vi "Target Get Gaussian Torque Setpoint.vi"(11 "Phase":dbl) -> (3 "Setpoint":dbl)   [LabVIEW 2018, in "COBRA Torque Setpoint Generators Library.lvlib"]
uses:
  COBRA Torque Setpoint Generators Library.lvlib
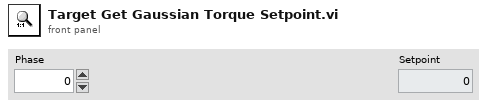
[diagram p1: front panel]
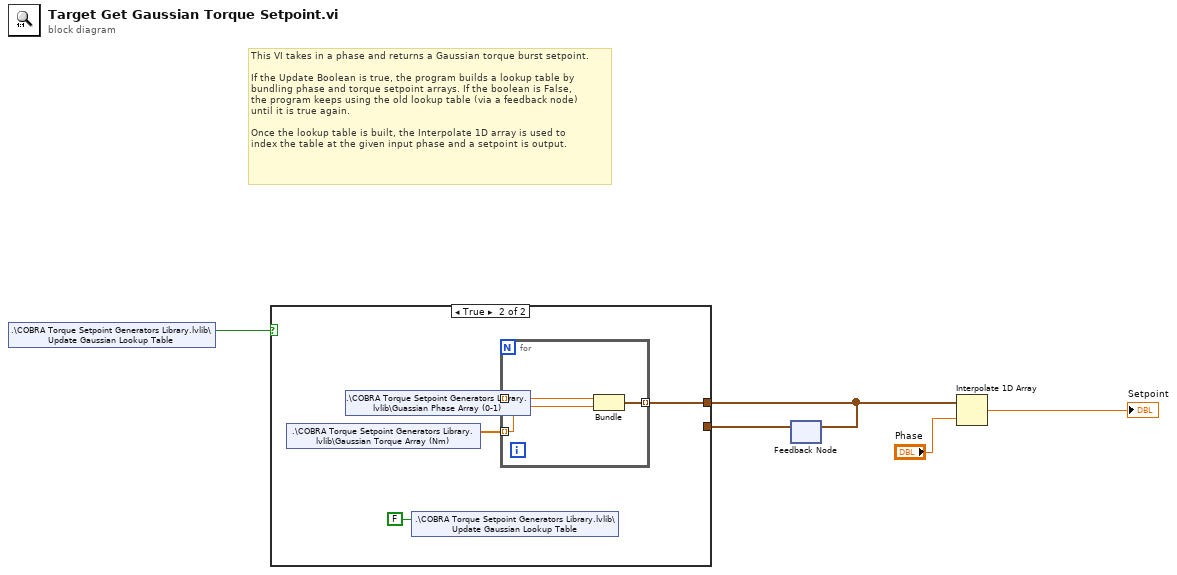
[diagram p0: block diagram]
diagram:
  # "This VI takes in a phase and returns a Gaussian torque burst setpoint.\n\nIf the Update Boolean is true, the program builds a lookup table by\nbundling phase and torque setpoint arrays. If the boolean is False, \nthe program keeps using the old lookup table (via a feedback node)\nuntil it is true again. \n\nOnce the lookup table is built, the Interpolate 1D array is used to\nindex the table at the given input phase and a setpoint is output."
  n1 = shared-variable ".\\COBRA Torque Setpoint Generators Library.lvlib\\Update Gaussian Lookup Table"() -> (w1:bool)  [unwired: 1 in, 1 out]
  n2 = feedback #1() -> (w5:cluster{"Numeric":dbl, "Numeric":dbl}[])  [unwired: 1 in]
  n3 = case shown="True" w1 {
    tunnel: [w6 w10] -> w4
    tunnel: w5 -> [w6 _]
    frame False {
    }
    frame True {
      n4 = shared-variable ".\\COBRA Torque Setpoint Generators Library.lvlib\\Gaussian Torque Array (Nm)"() -> (w8:dbl[])  [unwired: 1 in, 1 out]
      n5 = shared-variable ".\\COBRA Torque Setpoint Generators Library.lvlib\\Guassian Phase Array (0-1)"() -> (w9:dbl[])  [unwired: 1 in, 1 out]
      n6 = shared-variable ".\\COBRA Torque Setpoint Generators Library.lvlib\\Update Gaussian Lookup Table"(FALSE ("Update Gaussian Lookup Table")) -> ()  [unwired: 1 in, 1 out]
      n7 = for {
        tunnel: w9 -> [w13] mode=indexing
        tunnel: w8 -> [w12] mode=indexing
        tunnel: [w11] -> w10 mode=indexing
        n8 = Bundle("Numeric"=w13, "Numeric"=w12) -> (w11:cluster{"Numeric":dbl, "Numeric":dbl})  [unwired: 1 in]
      }
    }
  }
  n9 = feedback-in #1(w4) -> ()
  n10 = Interpolate 1D Array(1:"Phase", 2:w4) -> (0:→"Setpoint":dbl)
